vi "Initialise.vi"(8 "error in (no error)":errorcluster, 11 "File Sink in":refnum<class "File Sink.lvclass">) -> (0 "error out":errorcluster, 3 "File Sink out":refnum<class "File Sink.lvclass">)   [LabVIEW 2020, in "LV Log.lvlib" / "File Sink.lvclass"]
uses:
  File Sink.lvclass
  File Sink.lvclass/File Sink.ctl
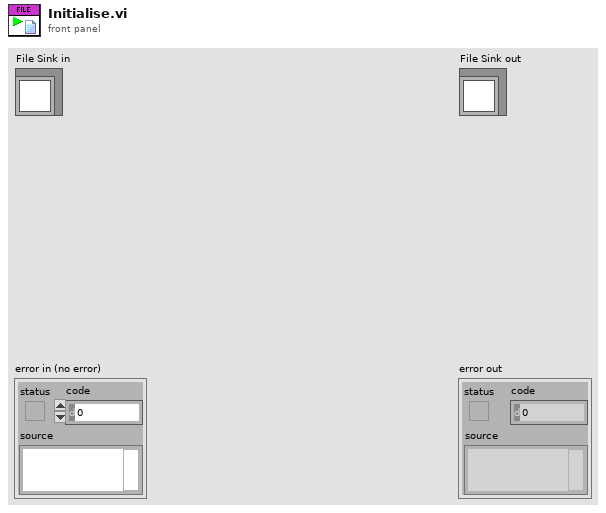
[diagram p1: front panel]
types:
  T1 = enum16{"open", "replace", "create", "open or create", "replace or create", "replace or create with confirmation"}
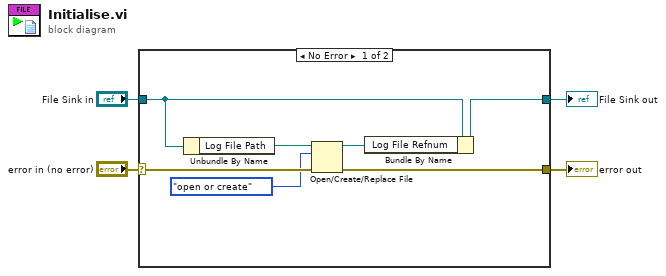
[diagram p0: block diagram]
diagram:
  n1 = case shown="No Error" "error in (no error)" {
    selector: "error in (no error)" -> [w10 w13]
    tunnel: [w9 w13] -> w3
    tunnel: "File Sink in" -> [w7 w12]
    tunnel: [w6 w12] -> w1
    frame No Error {
      n2 = Unbundle By Name(w7) -> ("Log File Path"=w11:path)
      n3 = Open/Create/Replace File(file path (use dialog)=w11, error in=w10, operation (0:open)=T1."open or create") -> (refnum out=w5:refnum<file>, error out=w9:errorcluster)  [unwired: 3 in, 1 out]
      n4 = Bundle By Name(cluster=w7, "Log File Refnum"=w5) -> (w6:refnum<class "File Sink.lvclass">)
    }
    frame Error {
    }
  }
  "error out" <- w3
  "File Sink out" <- w1
